vi "camera-startup.vi"() -> ()   [LabVIEW 2014]
doc: "Cools down the camera to operating temperature before use and returns it to ambient after use. Run this VI before running any other camera programs and leave it running the whole time you use the camera. To start: run vi, set temperature, check \"cooling\". To finish: Click \"warm up CCD and turn off camera\". Leave running until the program tells you that it has turned off the camera."
uses:
  SubVIs/Globals/Initilize Globals.vi
  SubVIs/Globals/Andor Camera Temperature.vi
  Library Files - Andor and MadCity/Andorlib/atmcd32d.lvlib
panel:
  in  "Temp. Set Point":i32(slide)=-70 scale=-120.0..20.0
  in  "Cooling":bool
  in  "Warm up CCD & Turn Off Camera":bool
  out "Cooling status":T1
  out "Detector Temperature":i32(graph)
  out "Camera Properties":T2
  out "Status":string
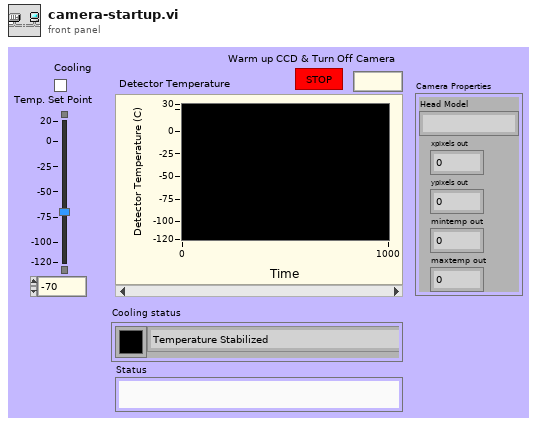
[diagram p1: front panel]
types:
  T1 = cluster{"Color Box":u32, "Cooling Status":enum16{"Temperature Stabilized", "Waiting to Stabilize Temperature", "Cooling is Turned Off", "Have not yet Reached Set Temperature"}}
  T2 = cluster{"Head Model":string, "xpixels out":i32, "ypixels out":i32, "mintemp out":i32, "maxtemp out":i32}
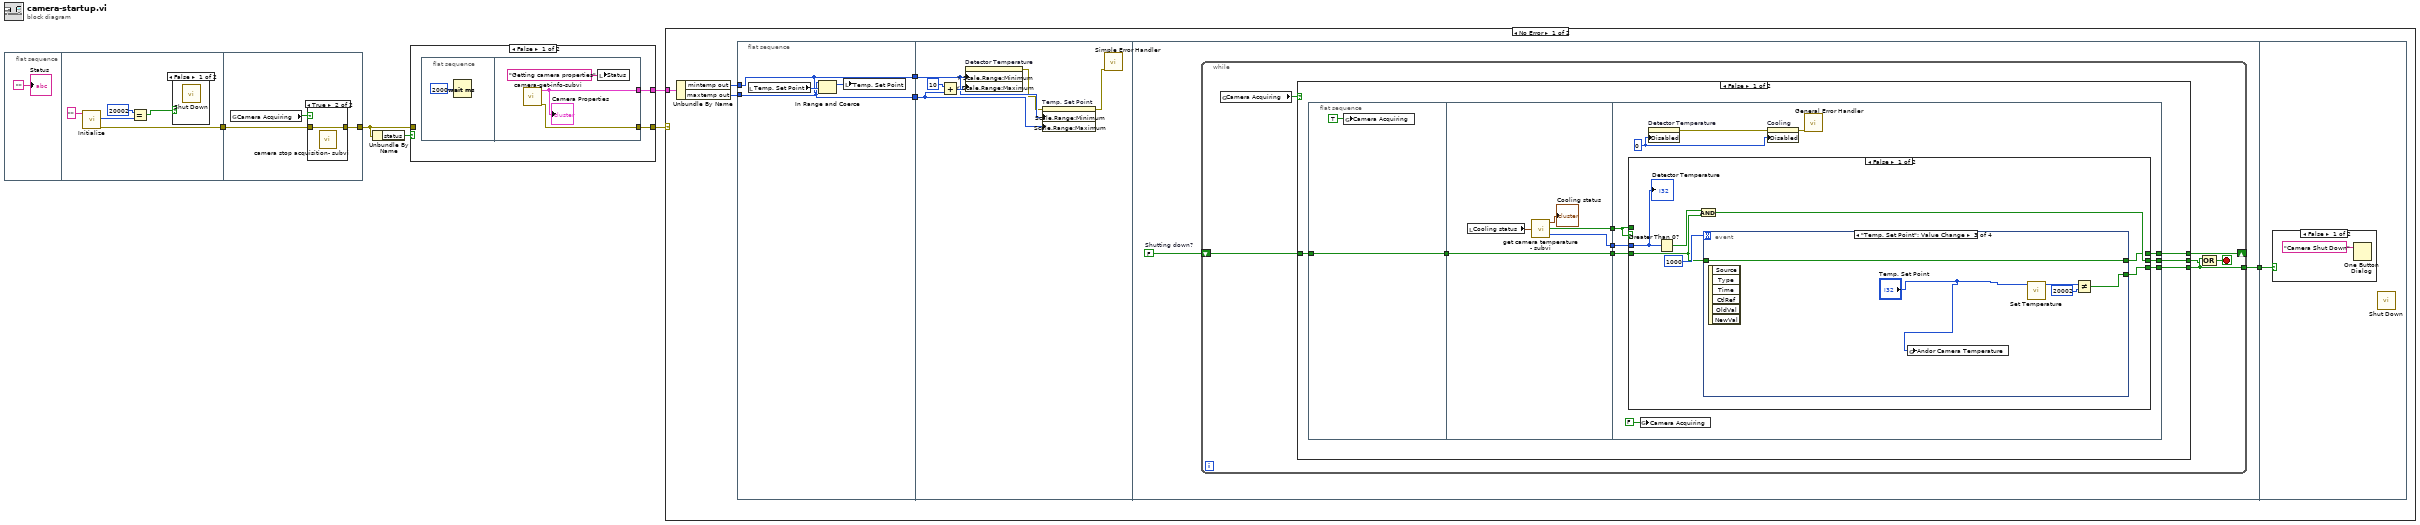
[diagram p0: block diagram]
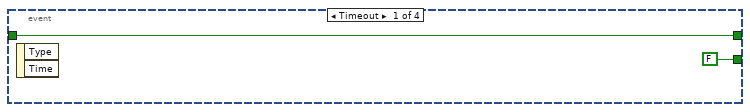
[diagram p2: hidden frame]
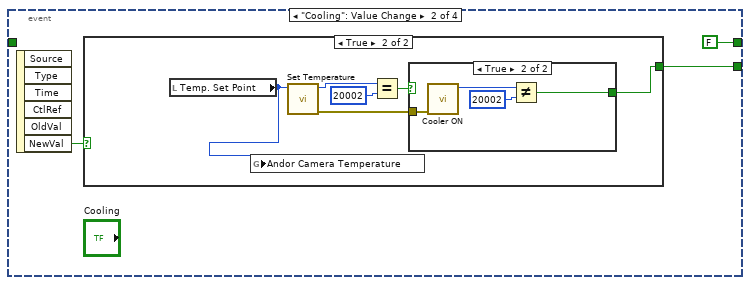
[diagram p3: hidden frame]
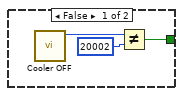
[diagram p4: hidden frame]
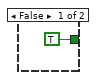
[diagram p5: hidden frame]
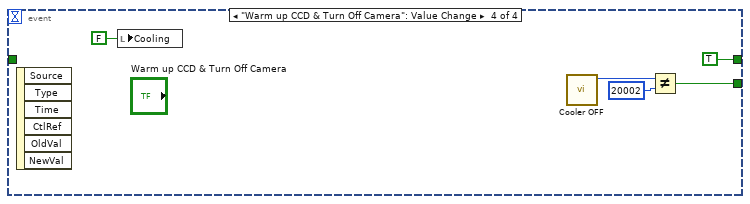
[diagram p6: hidden frame]
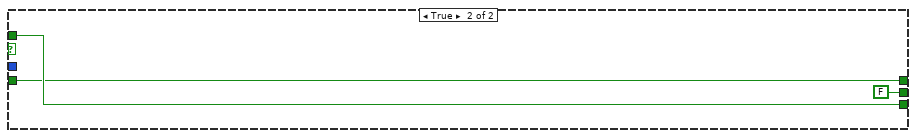
[diagram p7: hidden frame]
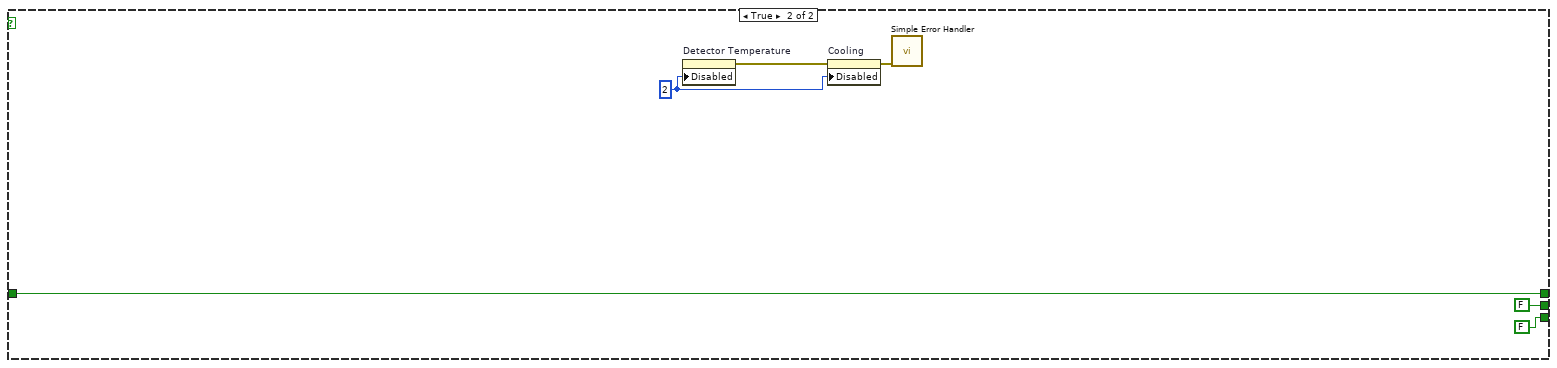
[diagram p8: hidden frame]
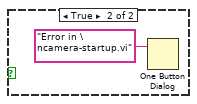
[diagram p9: hidden frame]
diagram:
  n1 = flat-sequence {
    tunnel: [w10] -> w5
    tunnel: w5 -> [w13]
    tunnel: [w12] -> w3
    frame #0 {
      "Status" <- ""
    }
    frame #1 {
      n2 = call "Initialize.vi"("dir"="") -> ("error out"=w10:errorcluster, "function return"=w9:u32)  [unwired: 8 in, 1 out]
      n3 = Equal?(x=u32 20002, y=w9) -> (x = y?=w7:bool)
      n4 = case shown="False" w7 {
        frame False {
          n5 = call "Shut Down.vi"() -> ()  [unwired: 10 in, 2 out]
        }
        frame True {
        }
      }
    }
    frame #2 {
      n6 = global read "Initilize Globals.vi" "Camera Acquiring"() -> (w14:bool)
      n7 = case shown="True" w14 {
        tunnel: [w15 w16] -> w12
        tunnel: w13 -> [w15 w16]
        frame False {
        }
        frame True {
          n8 = call "camera stop acquisition- subvi.vi"() -> ()  [unwired: 1 in]
        }
      }
    }
  }
  n9 = Unbundle By Name(w3) -> ("status"=w4:bool)
  n10 = case shown="False" w4 {
    tunnel: w3 -> [_ w23]
    tunnel: [w18 w23] -> w2
    tunnel: [w17 _] -> w1
    frame False {
      n11 = flat-sequence {
        tunnel: [w21] -> w18
        tunnel: [w20] -> w17
        frame #0 {
          n12 = Wait (ms)(milliseconds to wait=u32 2000) -> ()  [unwired: 1 out]
        }
        frame #1 {
          n13 = call "camera-get-info-subvi.vi"() -> ("error out"=w21:errorcluster, "Camera Properties"=w20:T2)  [unwired: 10 in]
          "Camera Properties" <- w20
          n14 = local write "Status"("Getting camera properties" ("Status")) -> ()
        }
      }
    }
    frame True {
    }
  }
  n15 = case shown="No Error" w2 {
    tunnel: w1 -> [w29 _]
    frame No Error {
      n16 = Unbundle By Name(w29) -> ("mintemp out"=w28:i32, "maxtemp out"=w27:i32)
      n17 = flat-sequence {
        tunnel: w28 -> [w30]
        tunnel: w27 -> [w31]
        tunnel: [w31] -> w26
        tunnel: [w30] -> w25
        tunnel: w26 -> [w35]
        tunnel: w25 -> [w36]
        tunnel: [w40] -> w24
        tunnel: w24 -> [w118]
        frame #0 {
          n18 = local read "Temp. Set Point"() -> (w33:i32)
          n19 = In Range and Coerce(upper limit=w31, x=w33, lower limit=w30) -> (coerced(x)=w32:i32)  [unwired: 1 out]
          n20 = local write "Temp. Set Point"(w32) -> ()
        }
        frame #1 {
          n21 = Add(x=10, y=w35) -> (x+y=w38:i32)
          n22 = property on="Detector Temperature" class="WFChart (strict)"("Y Scale.Range:Minimum"=w36, "Y Scale.Range:Maximum"=w38) -> (error out=w34:errorcluster)  [unwired: 2 in, 1 out]
          n23 = property on="Temp. Set Point" class="Slide (strict)"(error in=w34, "Scale.Range:Minimum"=w36, "Scale.Range:Maximum"=w35) -> (error out=w37:errorcluster)  [unwired: 1 in, 1 out]
          n24 = call <vilib>:"Simple Error Handler.vi"("error in (no error)"=w37) -> ()  [unwired: 1 in, 8 out]
        }
        frame #2 {
          w41 = FALSE  # Shutting down?
          n25 = while {
            shift-right: [w45] -> _
            shift-left: w41 -> [w46]
            tunnel: [w44] -> w40
            stop <- w43 stop-if-true
            n26 = global read "Initilize Globals.vi" "Camera Acquiring"() -> (w47:bool)
            n27 = case shown="False" w47 {
              tunnel: w46 -> [w51 w116]
              tunnel: [w53 FALSE] -> w42
              tunnel: [w48 w116] -> w45
              tunnel: [w49 FALSE] -> w44
              frame False {
                n28 = flat-sequence {
                  tunnel: [w56] -> w52
                  tunnel: w51 -> [w56]
                  tunnel: [w60] -> w55
                  tunnel: [w59] -> w54
                  tunnel: w52 -> [w58]
                  tunnel: [w58] -> w50
                  tunnel: w54 -> [w71]
                  tunnel: w55 -> [w70]
                  tunnel: [w69] -> w53
                  tunnel: w50 -> [w68]
                  tunnel: [w64] -> w49
                  tunnel: [w63] -> w48
                  frame #0 {
                    n29 = global write "Initilize Globals.vi" "Camera Acquiring"(TRUE) -> ()
                  }
                  frame #1 {
                    n30 = local read "Cooling status"() -> (w62:T1)
                    n31 = call "get camera temperature - subvi.vi"("Cooling Status In"=w62) -> ("Cooling Status Out"=→"Cooling status":T1, "Error?"=w59:bool, "temperature out"=w60:i32)
                  }
                  frame #2 {
                    w67 = u8 0 ("Disabled")
                    n32 = case shown="False" w71 {
                      tunnel: w71 -> [_ w111]
                      tunnel: w70 -> [w78 _]
                      tunnel: [w74 w111] -> w64
                      tunnel: [w76 FALSE] -> w69
                      tunnel: w68 -> [w75 w109]
                      tunnel: [w73 w109] -> w63
                      frame False {
                        n33 = Greater Than 0?(x=w78) -> (x > 0?=w77:bool)
                        n34 = And(x=w77, y=w75) -> (x .and. y?=w76:bool)
                        n35 = event shown="[2] \"Temp. Set Point\": Value Change" {
                          selector: _ -> [_ _ _ _]
                          dyn-events: _ -> [_ _ _ _]
                          timeout: 1000 -> [_ _ _ _]
                          tunnel: w75 -> [w81 _ w103 _]
                          tunnel: [w81 FALSE w103 TRUE] -> w73
                          tunnel: [FALSE ("status") w83 w100 w104] -> w74
                          event Timeout {
                            n36 = event-data() -> ()  [unwired: 3 out]
                          }
                          event "Cooling": Value Change {
                            n37 = event-data() -> ("NewVal"=w82:bool)  [unwired: 6 out]
                            n38 = case shown="True" w82 {
                              tunnel: [w86 w90] -> w83
                              frame False {
                                n39 = call "Cooler OFF.vi"() -> ("function return"=w85:u32)  [unwired: 10 in, 1 out]
                                n40 = Not Equal?(x=w85, y=20002) -> (x != y?=w86:bool)
                              }
                              frame True {
                                n41 = local read "Temp. Set Point"() -> (w88:i32)
                                n42 = global write "Andor Camera Temperature.vi" "Andor Camera Temperature"(w88) -> ()
                                n43 = call "Set Temperature.vi"("temperature"=w88) -> ("error out"=w89:errorcluster, "function return"=w92:u32)  [unwired: 9 in]
                                n44 = Equal?(x=w92, y=20002) -> (x = y?=w93:bool)
                                n45 = case shown="True" w93 {
                                tunnel: [TRUE w95] -> w90
                                tunnel: w89 -> [_ w98]
                                frame False {
                                }
                                frame True {
                                n46 = call "Cooler ON.vi"("error in (no error)"=w98) -> ("function return"=w96:u32)  [unwired: 9 in, 1 out]
                                n47 = Not Equal?(x=w96, y=20002) -> (x != y?=w95:bool)
                                }
                                }
                              }
                            }
                          }
                          event "Temp. Set Point": Value Change {
                            n48 = event-data() -> ()  [unwired: 7 out]
                            n49 = global write "Andor Camera Temperature.vi" "Andor Camera Temperature"("Temp. Set Point") -> ()
                            n50 = call "Set Temperature.vi"("temperature"="Temp. Set Point") -> ("function return"=w101:u32)  [unwired: 9 in, 1 out]
                            n51 = Not Equal?(x=w101, y=20002) -> (x != y?=w100:bool)
                          }
                          event "Warm up CCD & Turn Off Camera": Value Change {
                            n52 = event-data() -> ()  [unwired: 7 out]
                            n53 = local write "Cooling"(FALSE ("Cooling")) -> ()
                            n54 = call "Cooler OFF.vi"() -> ("function return"=w105:u32)  [unwired: 10 in, 1 out]
                            n55 = Not Equal?(x=w105, y=20002) -> (x != y?=w104:bool)
                          }
                        }
                        "Detector Temperature" <- w78
                      }
                      frame True {
                      }
                    }
                    n56 = global write "Initilize Globals.vi" "Camera Acquiring"(FALSE) -> ()
                    n57 = property on="Detector Temperature" class="WFChart (strict)"("Disabled"=w67) -> (error out=w66:errorcluster)  [unwired: 2 in, 1 out]
                    n58 = property on="Cooling" class="Bool (strict)"(error in=w66, "Disabled"=w67) -> (error out=w65:errorcluster)  [unwired: 1 in, 1 out]
                    n59 = call <vilib>:"General Error Handler.vi"("error in (no error)"=w65) -> ()  [unwired: 10 in, 5 out]
                  }
                }
              }
              frame True {
                w114 = u8 2 ("Disabled")
                n60 = property on="Detector Temperature" class="WFChart (strict)"("Disabled"=w114) -> (error out=w113:errorcluster)  [unwired: 2 in, 1 out]
                n61 = property on="Cooling" class="Bool (strict)"(error in=w113, "Disabled"=w114) -> (error out=w112:errorcluster)  [unwired: 1 in, 1 out]
                n62 = call <vilib>:"Simple Error Handler.vi"("error in (no error)"=w112) -> ()  [unwired: 1 in, 8 out]
              }
            }
            n63 = Compound Arithmetic op=OR(w44, w42) -> (w43:bool)
          }
        }
        frame #3 {
          n64 = case shown="False" w118 {
            frame False {
              n65 = One Button Dialog(message="Camera Shut Down" ("string")) -> ()  [unwired: 2 out]
            }
            frame True {
              n66 = One Button Dialog(message="Error in \ncamera-startup.vi" ("string")) -> ()  [unwired: 2 out]
            }
          }
          n67 = call "Shut Down.vi"() -> ()  [unwired: 10 in, 2 out]
        }
      }
    }
    frame Error {
    }
  }
